vi "Read controller_.vi"(8 "error in (no error)":errorcluster, 11 "Configurable Device in":refnum<class "Configurable Device.lvclass">) -> (0 "error out":errorcluster, 2 "controller?":bool, 3 "Configurable Device out":refnum<class "Configurable Device.lvclass">)   [LabVIEW 2014, in "Device.lvlib" / "Configurable Device.lvclass"]
uses:
  Configurable Device.lvclass
  Configurable Device.lvclass/Configurable Device.ctl
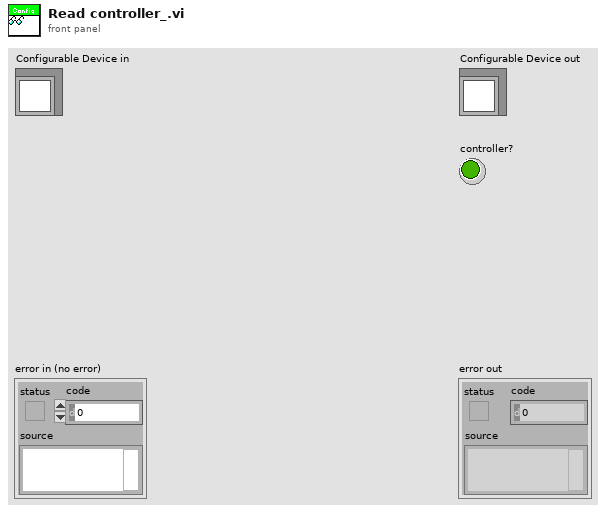
[diagram p1: front panel]
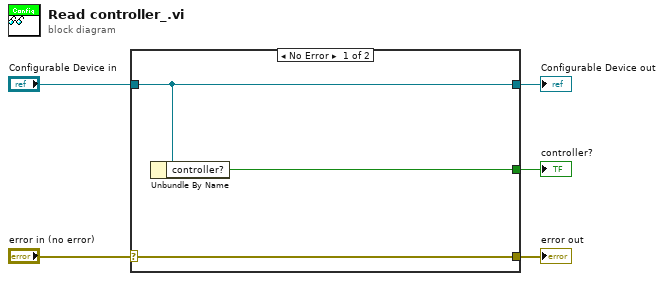
[diagram p0: block diagram]
diagram:
  n1 = case shown="No Error" "error in (no error)" {
    selector: "error in (no error)" -> [w8 w9]
    tunnel: [w8 w9] -> w4
    tunnel: [w7 w10] -> w2
    tunnel: "Configurable Device in" -> [w7 w10]
    tunnel: [w6 _] -> w1
    frame No Error {
      n2 = Unbundle By Name(w7) -> ("controller?"=w6:bool)
    }
    frame Error {
    }
  }
  "error out" <- w4
  "Configurable Device out" <- w2
  "controller?" <- w1
